vi "CRYCheck Main Receiver.vi"(11 "Rcv Idx":i32) -> (3 "Is Main?":bool)   [LabVIEW 2013]
uses:
  CRYMisc vis settings global.vi
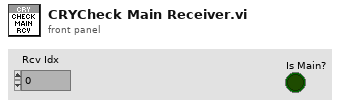
[diagram p1: front panel]
types:
  T1 = cluster{"Rcv Idx":i32, "Chn Idx":i32, "Data":i32[], "bufCount":i32}[]
  T2 = cluster{"Rcv Idx":i32, "Chn Idx":i32, "Data":i32[], "bufCount":i32}
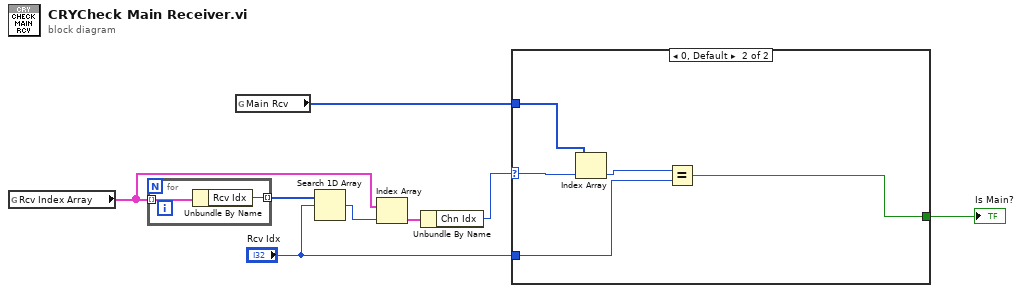
[diagram p0: block diagram]
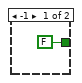
[diagram p2: hidden frame]
diagram:
  n1 = global read "CRYMisc vis settings global.vi" "Rcv Index Array"() -> (w3:T1)
  n2 = for {
    tunnel: w3 -> [w10] mode=indexing
    tunnel: [w9] -> w6 mode=indexing
    n3 = Unbundle By Name(w10) -> ("Rcv Idx"=w9:i32)
  }
  n4 = global read "CRYMisc vis settings global.vi" "Main Rcv"() -> (w7:i32[])
  n5 = Search 1D Array(1D array=w6, element="Rcv Idx") -> (index of element=w4:i32)  [unwired: 1 in]
  n6 = Index Array(array=w3, index=w4) -> (element=w2:T2)
  n7 = Unbundle By Name(w2) -> ("Chn Idx"=w1:i32)
  n8 = case shown="0, Default" w1 {
    selector: w1 -> [_ w12]
    tunnel: [FALSE w15] -> w8
    tunnel: w7 -> [_ w14]
    tunnel: "Rcv Idx" -> [_ w13]
    frame -1 {
    }
    frame 0, Default {
      n9 = Index Array(array=w14, index=w12) -> (element=w16:i32)
      n10 = Equal?(x=w16, y=w13) -> (x = y?=w15:bool)
    }
  }
  "Is Main?" <- w8
